vi "configure.vi"(8 "error in (no error)":errorcluster, 11 "SignalReaderCN091129DAQmx in":refnum<class "SignalReaderCN091129DAQmx.lvclass">) -> (0 "error out":errorcluster, 3 "SignalReaderCN091129DAQmx out":refnum<class "SignalReaderCN091129DAQmx.lvclass">)   [LabVIEW 2010, in "SignalReaderCN091129DAQmx.lvclass"]
doc: "The dynamic dispatch version of this VI loads and displays the configuration file associated with the plug-in object. The user modify and save the configuration data."
uses:
  SignalReaderCN091129DAQmx.lvclass
  SignalReaderCN091129DAQmx.lvclass/SignalReaderCN091129DAQmx.ctl
  common/classes/GenericComponent/GenericComponent/GenericComponent.lvclass
panel:
  in  "clock Source":tag
  in  "time-out":dbl[unit]=0.5
  in  "maximum sampling rate":dbl[unit]
  in  "remove":bool
  in  "edit":bool
  in  "Add":bool
  in  "Analog Input Channels":i32(listbox)
  out "configuration":string
  in  "cancel":bool
  in  "save":bool
  # "Configure CN091129DAQmxReadSignals"
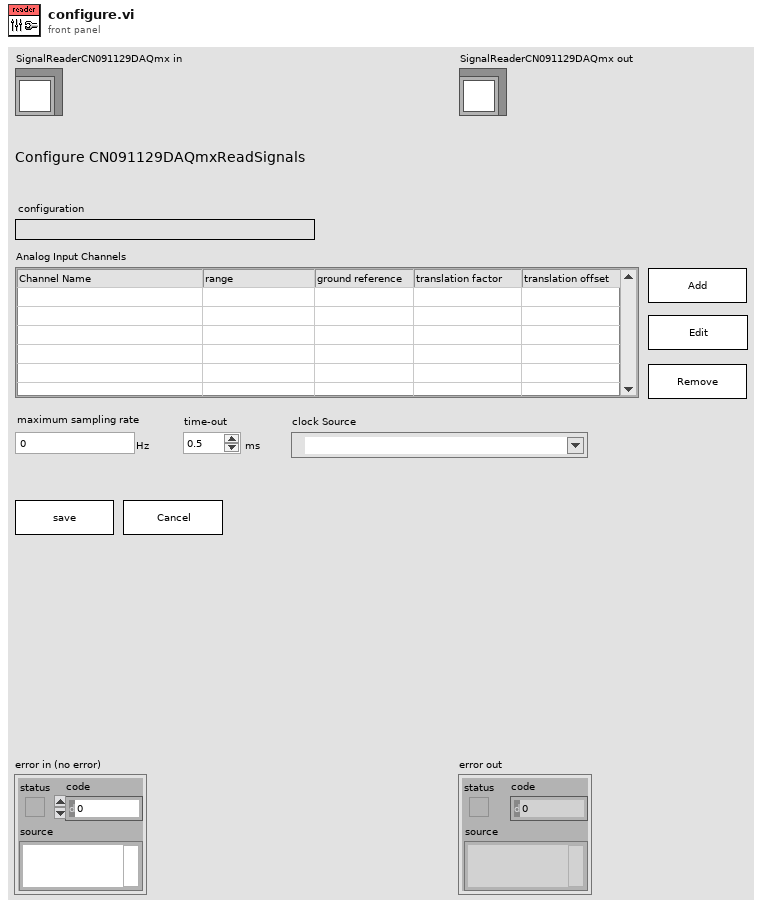
[diagram p1: front panel]
types:
  T1 = typedef "SignalReaderCN091129DAQmx.lvclass/channel_definition_cluster.ctl" = cluster{"physical Channel":string, "max_input_value":dbl, "min_input_value":dbl, "ground_reference":i32, "translation_factor":dbl, "translation_offset":dbl}
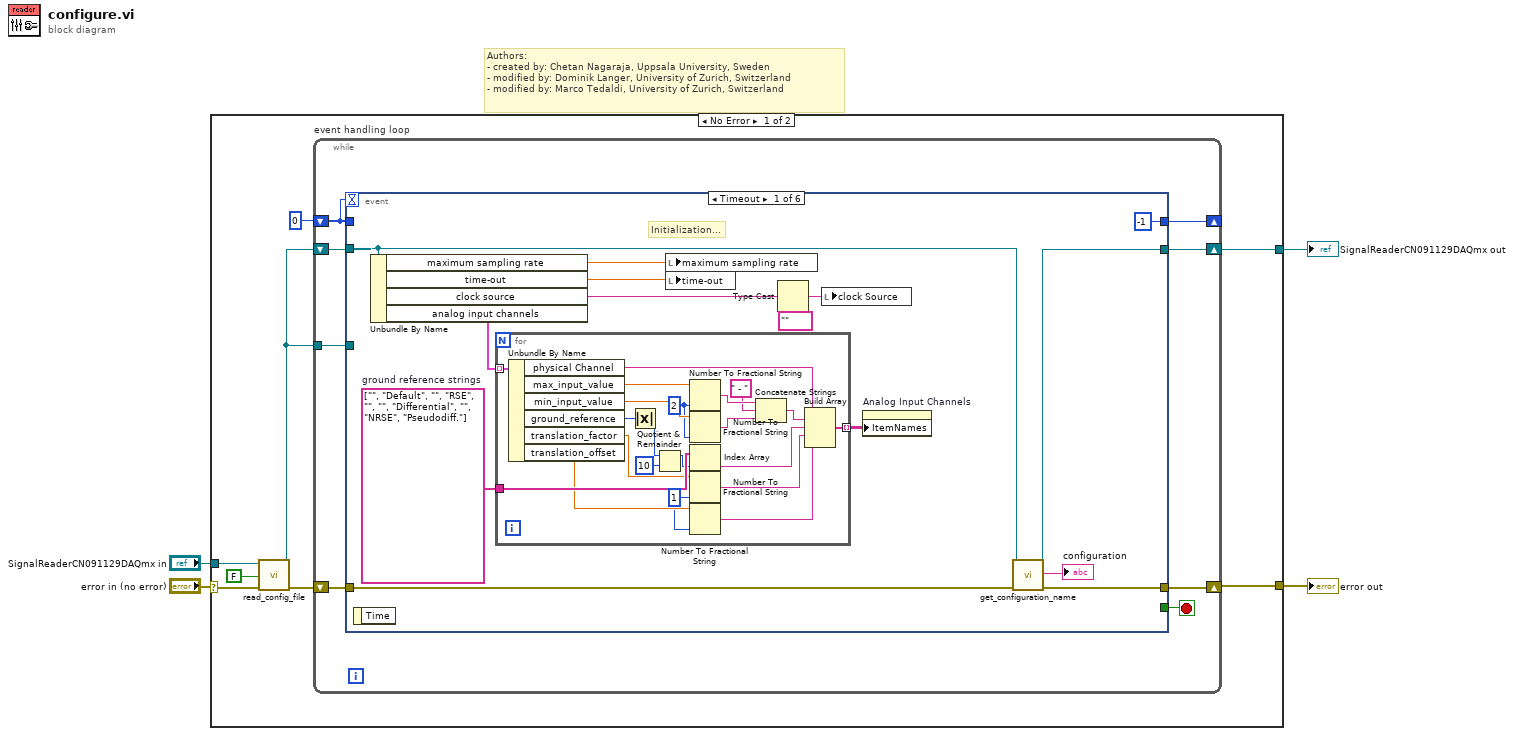
[diagram p0: block diagram]
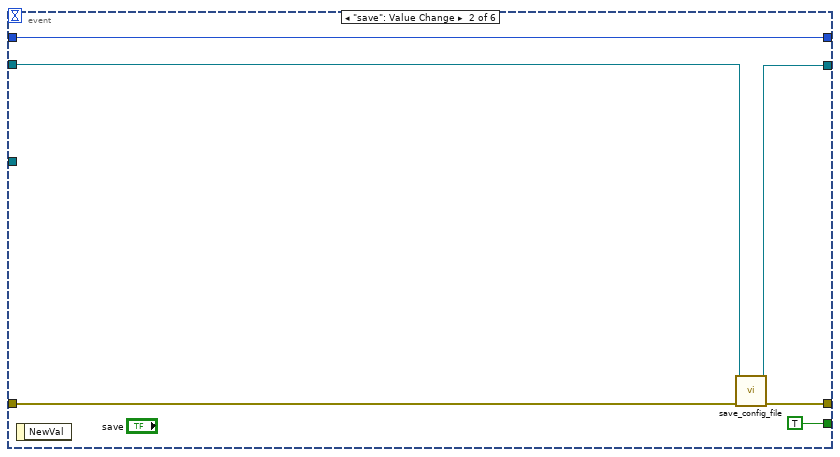
[diagram p2: hidden frame]
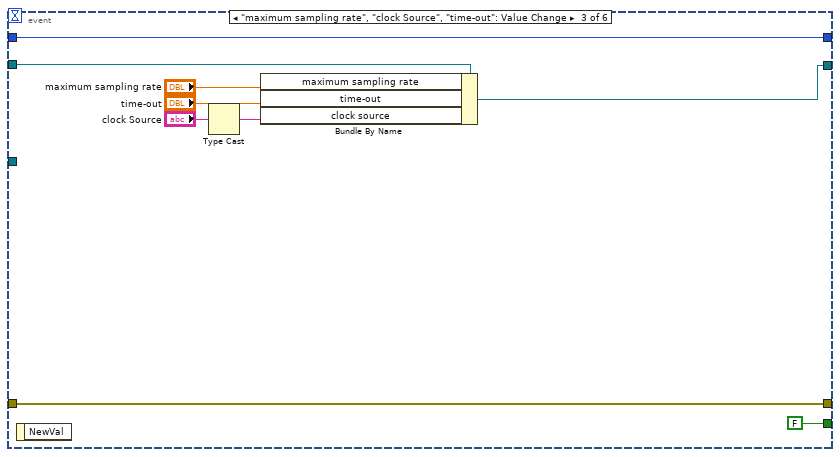
[diagram p3: hidden frame]
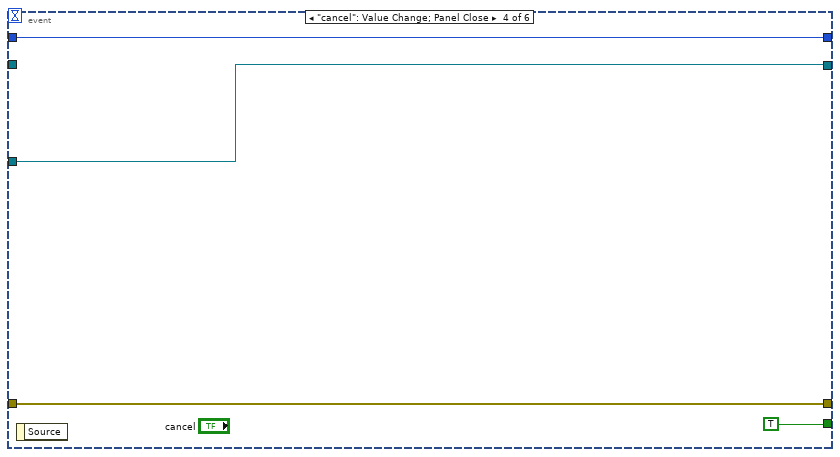
[diagram p4: hidden frame]
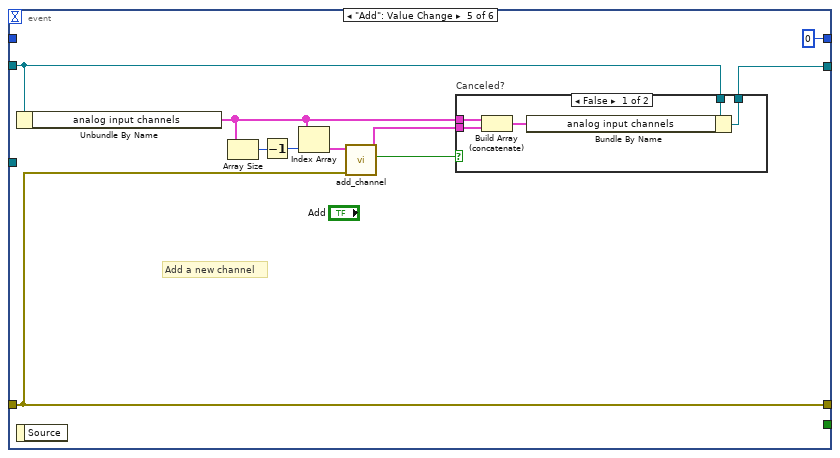
[diagram p5: hidden frame]
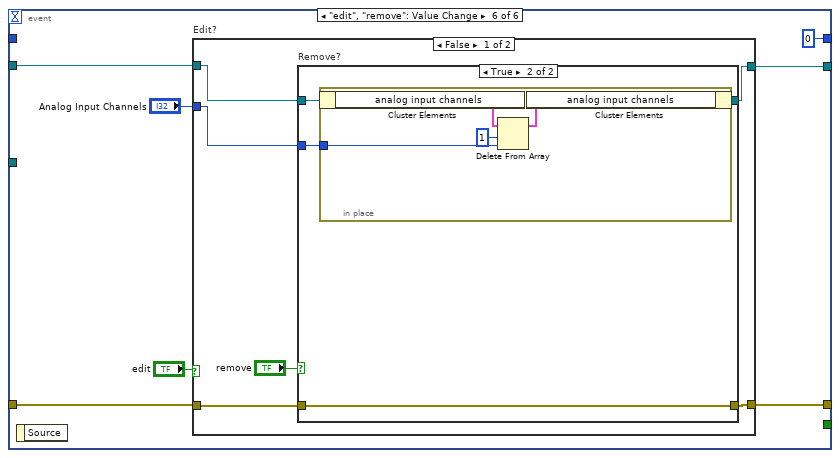
[diagram p7: hidden frame]
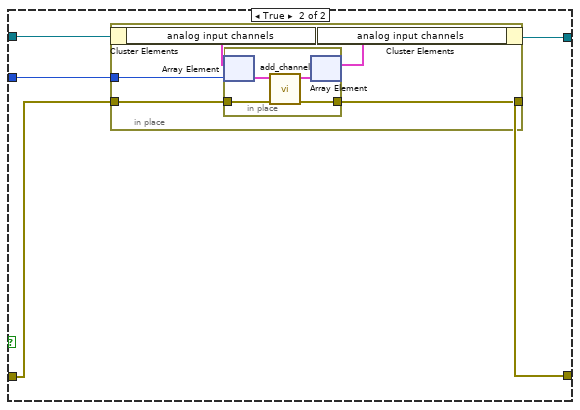
[diagram p9: hidden frame]
diagram:
  # "Authors: \n- created by: Chetan Nagaraja, Uppsala University, Sweden\n- modified by: Dominik Langer, University of Zurich, Switzerland\n- modified by: Marco Tedaldi, University of Zurich, Switzerland"
  n1 = case shown="No Error" "error in (no error)" {
    selector: "error in (no error)" -> [w11 w128]
    tunnel: "SignalReaderCN091129DAQmx in" -> [w12 w129]
    tunnel: [w6 w129] -> w4
    tunnel: [w8 w128] -> w3
    frame No Error {
      n2 = call-dynamic "read_config_file.vi"("error in (no error)"=w11, "force load?"=FALSE, "GenericPlugin in"=w12) -> ("error out"=w9:errorcluster, "GenericPlugin out"=w5:refnum<class "SignalReaderCN091129DAQmx.lvclass">)  [unwired: 7 in]
      n3 = while "event handling loop" {
        shift-right: [w17] -> _
        shift-left: 0 -> [w15]
        shift-right: [w16] -> w6
        shift-left: w5 -> [w14]
        shift-right: [w18] -> w8
        shift-left: w9 -> [w19]
        tunnel: w5 -> [w13]
        stop <- w20 stop-if-true
        n4 = event shown="[0] Timeout" {
          selector: _ -> [_ _ _ _ _ _]
          dyn-events: _ -> [_ _ _ _ _ _]
          timeout: w15 -> [_ _ _ _ _ _]
          tunnel: [_ TRUE FALSE TRUE _ _] -> w20
          tunnel: w19 -> [w26 w57 w63 w74 w84 w92]
          tunnel: w14 -> [w30 w56 w68 _ w76 w94]
          tunnel: [w31 w60 w62 w71 w75 w95] -> w16
          tunnel: [w33 w59 w63 w74 w84 w91] -> w18
          tunnel: w15 -> [_ w58 w69 w72 _ _]
          tunnel: [-1 w58 w69 w72 0 0] -> w17
          tunnel: w13 -> [_ _ _ w71 _ _]
          event Timeout {
            w21 = string[] ["", "Default", "", "RSE", "", "", "Differential", "", "NRSE", "Pseudodiff."]  # ground reference strings
            # "Initialization..."
            n5 = event-data() -> ()  [unwired: 1 in, 1 out]
            n6 = Unbundle By Name(w30) -> ("maximum sampling rate"=w27:dbl[unit], "time-out"=w22:dbl[unit], "clock source"=w29:string, "analog input channels"=w25:T1[])
            n7 = for {
              tunnel: w25 -> [w55] mode=indexing
              tunnel: w21 -> [w52]
              tunnel: [w40] -> w24 mode=indexing
              w48 = i16 1 ("precision (6)")
              w49 = i16 2 ("precision (6)")
              n8 = Unbundle By Name(w55) -> ("physical Channel"=w39:string, "max_input_value"=w54:dbl, "min_input_value"=w53:dbl, "ground_reference"=w36:i32, "translation_factor"=w51:dbl, "translation_offset"=w50:dbl)
              n9 = Absolute Value(x=w36) -> (abs(x)=w35:i32)
              n10 = Quotient & Remainder(x=w35, y=10) -> (x-y*floor(x/y)=w38:i32)  [unwired: 1 out]
              n11 = Number To Fractional String(number=w54, precision (6)=w49) -> (F-format string=w47:string)  [unwired: 2 in]
              n12 = Number To Fractional String(number=w53, precision (6)=w49) -> (F-format string=w46:string)  [unwired: 2 in]
              n13 = Index Array(array=w52, index=w38) -> (element=w43:string)
              n14 = Number To Fractional String(number=w51, precision (6)=w48) -> (F-format string=w42:string)  [unwired: 2 in]
              n15 = Number To Fractional String(number=w50, precision (6)=w48) -> (F-format string=w41:string)  [unwired: 2 in]
              n16 = Concatenate Strings(w47, " - " ("string"), w46) -> (w44:string)
              n17 = Build Array(w39, w44, w43, w42, w41) -> (w40:string[])
            }
            n18 = local write "maximum sampling rate"(w27) -> ()
            n19 = local write "time-out"(w22) -> ()
            n20 = Type Cast(type=tag "" ("clock Source"), x=w29) -> (*(type *) &x=w23:tag)
            n21 = local write "clock Source"(w23) -> ()
            n22 = property on="Analog Input Channels" class="MCListbox (strict)"("ItemNames"=w24) -> ()  [unwired: 2 in, 2 out]
            n23 = call "get_configuration_name.vi"("error in (no error)"=w26, "GenericPlugin.lvclass in"=w30) -> ("error out"=w33:errorcluster, "configuration name"=→"configuration":string, "GenericPlugin.lvclass out"=w31:refnum<class "SignalReaderCN091129DAQmx.lvclass">)  [unwired: 7 in]
          }
          event "save": Value Change {
            n24 = event-data() -> ()  [unwired: 1 in, 1 out]
            n25 = call-dynamic "save_config_file.vi"("error in (no error)"=w57, "GenericPlugin in"=w56) -> ("error out"=w59:errorcluster, "GenericPlugin out"=w60:refnum<class "SignalReaderCN091129DAQmx.lvclass">)  [unwired: 2 in, 6 out]
          }
          event "maximum sampling rate", "clock Source", "time-out": Value Change {
            n26 = event-data() -> ()  [unwired: 1 in, 1 out]
            n27 = Type Cast(x="clock Source") -> (*(type *) &x=w66:string)  [unwired: 1 in]
            n28 = Bundle By Name(cluster=w68, "maximum sampling rate"="maximum sampling rate", "time-out"="time-out", "clock source"=w66) -> (w62:refnum<class "SignalReaderCN091129DAQmx.lvclass">)
          }
          event "cancel": Value Change; Panel Close {
            n29 = event-data() -> ()  [unwired: 1 in, 1 out]
          }
          event "Add": Value Change {
            # "Add a new channel"
            n30 = Unbundle By Name(w76) -> ("analog input channels"=w79:T1[])
            n31 = event-data() -> ()  [unwired: 1 in, 1 out]
            n32 = Array Size(array=w79) -> (size(s)=w83:i32)
            n33 = Decrement(x=w83) -> (x-1=w82:i32)
            n34 = Index Array(array=w79, index=w82) -> (element=w81:T1)
            n35 = call "add_channel.vi"("error in (no error)"=w84, "Channel definition in"=w81) -> ("Canceled"=w78:bool, "Channel definition out"=w80:T1)  [unwired: 7 in, 1 out]
            n36 = case "Canceled?" shown="False" w78 {
              tunnel: w80 -> [w89 _]
              tunnel: w79 -> [w88 _]
              tunnel: w76 -> [w86 w90]
              tunnel: [w85 w90] -> w75
              frame False {
                n37 = Build Array (concatenate)(w88, w89) -> (w87:T1[])
                n38 = Bundle By Name(cluster=w86, "analog input channels"=w87) -> (w85:refnum<class "SignalReaderCN091129DAQmx.lvclass">)
              }
              frame True {
              }
            }
          }
          event "edit", "remove": Value Change {
            n39 = event-data() -> ()  [unwired: 1 in, 1 out]
            n40 = case "Edit?" shown="False" "edit" {
              tunnel: [w99 w116] -> w95
              tunnel: w94 -> [w100 w117]
              tunnel: "Analog Input Channels" -> [w98 w118]
              tunnel: w92 -> [w101 w115]
              tunnel: [w102 w114] -> w91
              frame False {
                n41 = case "Remove?" shown="True" "remove" {
                  tunnel: [w105 w109] -> w102
                  tunnel: w101 -> [w105 w109]
                  tunnel: w100 -> [w104 w108]
                  tunnel: [w104 w107] -> w99
                  tunnel: w98 -> [_ w106]
                  frame False {
                    # "Thid should not happen. But just do nothing here."
                  }
                  frame True {
                    n42 = in-place {
                      in-place-border: w106 -> [w113]
                      n43 = in-place-cluster #1(w108) -> ("analog input channels"=w111:T1[])
                      n44 = Delete From Array(array=w111, length=1, index=w113) -> (array with subset deleted=w110:T1[])  [unwired: 1 out]
                      n45 = in-place-cluster #1("analog input channels"=w110) -> (w107:refnum<class "SignalReaderCN091129DAQmx.lvclass">)
                    }
                  }
                }
              }
              frame True {
                n46 = in-place {
                  in-place-border: w118 -> [w123]
                  in-place-border: w115 -> [w120]
                  in-place-border: [w119] -> w114
                  n47 = in-place-cluster #2(w117) -> ("analog input channels"=w122:T1[])
                  n48 = in-place {
                    in-place-border: w120 -> [w125]
                    in-place-border: [w124] -> w119
                    n49 = in-place-array #3(w122, w123) -> (w127:T1)
                    n50 = call "add_channel.vi"("error in (no error)"=w125, "Channel definition in"=w127) -> ("error out"=w124:errorcluster, "Channel definition out"=w126:T1)  [unwired: 7 in, 1 out]
                    n51 = in-place-array #3(w126) -> (w121:T1[])  [unwired: 1 out]
                  }
                  n52 = in-place-cluster #2("analog input channels"=w121) -> (w116:refnum<class "SignalReaderCN091129DAQmx.lvclass">)
                }
              }
            }
          }
        }
      }
    }
    frame Error {
    }
  }
  "error out" <- w3
  "SignalReaderCN091129DAQmx out" <- w4
